vi "Matrix Logarithm.vi"   [LabVIEW 2014, in "NI_AALBase.lvlib"]
doc: "Computes the natural logarithm of a square <B>Input Matrix</B>. Wire data to the <B>Input Matrix</B> input to determine the polymorphic instance to use or manually select the instance."
uses:
  NI_AALBase.lvlib
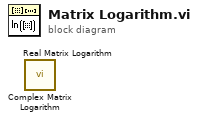
[diagram p0: block diagram]
diagram:
  n1 = call "Complex Matrix Logarithm.vi"() -> ()  [unwired: 2 in, 2 out]
  n2 = call "Real Matrix Logarithm.vi"() -> ()  [unwired: 2 in, 2 out]
